vi "log analysis_gps.vi"() -> ()   [LabVIEW 2019] (continued)
\tsystem status\tnormal 2 28.000000 0 0\trobot status\t300.742789\t57.868654\t10.465800\t0.003841\t1.974526\t-29.727465\t0.303000\t-0.016000\n\t\n15:24:51.1\tlog_raw\tgps_raw\t#INSPVAXA,USB3,0,50.0,FINESTEERING,2107,282309.100,02000000,471d,15824;INS_ALIGNMENT_COMPLETE,INS_RTKFIXED,37.37065087449,126.72423169405,10.4716,22.3000,-0.1818,0.2462,0.0157,-0.101661617,1.756669202,119.993193465,0.5316,0.3505,0.6792,0.1345,0.1096,0.0793,0.1439,0.1491,4.9301,0f000001,0*2fa2c19e\n\tsystem status\tnormal 2 28.000000 0 0\trobot status\t300.864286\t57.781823\t10.471600\t-0.101662\t1.756669\t-29.993193\t0.301000\t-0.019000\n\t\n15:24:51.6\tlog_raw\tgps_raw\t#INSPVAXA,USB3,0,50.5,FINESTEERING,2107,282309.600,02000000,471d,15824;INS_ALIGNMENT_COMPLETE,INS_RTKFIXED,37.37065005438,126.72423301384,10.4771,22.3000,-0.1715,0.2318,0.0129,-0.072761707,1.702932866,120.296688789,0.5316,0.3505,0.6792,0.1345,0.1096,0.0793,0.1439,0.1491,4.9301,0f000001,0*35eea818\n\tsystem status\tnormal 2 28.000000 0 0\trobot status\t300.981191\t57.690799\t10.477100\t-0.072762\t1.702933\t-30.296689\t0.299000\t-0.017000\n\t\n15:24:52.1\tlog_raw\tgps_raw\t#DUALANTENNAHEADINGA,USB3,0,50.0,FINESTEERING,2107,282310.100,02000000,d426,15824;INSUFFICIENT_OBS,NONE,0.000000000,0.000000000,0.000000000,0.0,0.000000000,0.000000000,\"\",0,0,0,0,00,00,00,00*14cc2e90\n\tsystem status\tnormal 2 28.000000 0 0\trobot status\t301.096541\t57.598411\t10.483200\t0.061278\t1.632933\t-30.590921\t0.298000\t-0.016000\n\t\n15:24:52.6\tlog_raw\tgps_raw\t#INSPVAXA,USB3,0,50.0,FINESTEERING,2107,282310.600,02000000,471d,15824;INS_ALIGNMENT_COMPLETE,INS_RTKFIXED,37.37064838288,126.72423565428,10.4879,22.3000,-0.1825,0.2221,0.0118,0.275691228,1.663027619,120.773343582,0.5316,0.3505,0.6792,0.1345,0.1096,0.0793,0.1439,0.1491,4.9301,0f000001,0*997564fa\n\tsystem status\tnormal 2 28.000000 0 0\trobot status\t301.215077\t57.505280\t10.487900\t0.275691\t1.663028\t-30.773344\t0.300000\t-0.012000\n\t\n15:24:53.1\tlog_raw\tgps_raw\t#DUALANTENNAHEADINGA,USB3,0,46.0,FINESTEERING,2107,282311.100,02000000,d426,15824;SOL_COMPUTED,NARROW_FLOAT,-1.000000000,117.813430786,-36.691406250,0.0,360.000000000,180.000000000,\"631T\",17,7,7,6,04,00,20,03*31d6dfd5\n\tsystem status\tnormal 2 28.000000 0 0\trobot status\t301.329857\t57.414343\t10.492200\t0.192572\t1.804077\t-31.004968\t0.300000\t-0.009000\n\t\n15:24:53.6\tlog_raw\tgps_raw\t#DUALANTENNAHEADINGA,USB3,0,46.0,FINESTEERING,2107,282311.600,02000000,d426,15824;SOL_COMPUTED,NARROW_FLOAT,-1.000000000,120.262771606,-39.374176025,0.0,360.000000000,180.000000000,\"631T\",18,7,7,5,04,00,20,03*970c933d\n\tsystem status\tnormal 2 28.000000 0 0\trobot status\t301.442602\t57.321734\t10.497200\t0.226704\t1.873089\t-31.248181\t0.301000\t-0.010000\n\t\n15:24:54.1\tlog_raw\tgps_raw\t#INSPVAXA,USB3,0,48.5,FINESTEERING,2107,282312.100,02000000,471d,15824;INS_ALIGNMENT_COMPLETE,INS_RTKFIXED,37.37064587490,126.72423949786,10.5026,22.3000,-0.1922,0.2292,0.0073,0.477048241,1.745843480,121.477542384,0.5806,0.3850,0.7206,0.1397,0.1125,0.0814,0.1439,0.1495,4.9286,0f000001,0*cdf8ddfc\n\tsystem status\tnormal 2 28.000000 0 0\trobot status\t301.555535\t57.226921\t10.502600\t0.477048\t1.745843\t-31.477542\t0.299000\t-0.001000\n\t\n15:24:54.6\tlog_raw\tgps_raw\t#DUALANTENNAHEADINGA,USB3,0,48.5,FINESTEERING,2107,282312.600,02000000,d426,15824;INSUFFICIENT_OBS,NONE,0.000000000,0.000000000,0.000000000,0.0,0.000000000,0.000000000,\"\",0,0,0,0,00,00,00,00*914fc627\n\tsystem status\tnormal 2 28.100000 0 0\trobot status\t301.668360\t57.139659\t10.506800\t0.443490\t1.749413\t-31.695525\t0.299000\t0.005000\n\t\n15:24:55.1\tlog_raw\tgps_raw\t#INSPVAXA,USB3,0,48.0,FINESTEERING,2107,282313.100,02000000,471d,15824;INS_ALIGNMENT_COMPLETE,INS_RTKFIXED,37.37064429153,126.72424202455,10.5097,22.3000,-0.1991,0.2355,-0.0061,0.301334832,1.691394524,121.905200566,0.5806,0.3850,0.7206,0.1397,0.1125,0.0814,0.1439,0.1495,4.9286,0f000001,0*1a642130\n\tsystem status\tnormal 2 28.100000 0 0\trobot status\t301.779345\t57.051183\t10.509700\t0.301335\t1.691395\t-31.905201\t0.295000\t0.004000\n\t\n15:24:55.6\tlog_raw\tgps_raw\t#DUALANTENNAHEADINGA,USB3,0,48.0,FINESTEERING,2107,282313.600,02000000,d426,15824;INSUFFICIENT_OBS,NONE,0.000000000,0.000000000,0.000000000,0.0,0.000000000,0.000000000,\"\",0,0,0,0,00,00,00,00*80ae0999\n\tsystem status\tnormal 2 28.100000 0 0\trobot status\t301.892959\t56.952693\t10.513100\t0.176842\t1.740351\t-31.947906\t0.299000\t0.002000\n\t\n15:24:56.1\tlog_raw\tgps_raw\t#DUALANTENNAHEADINGA,USB3,0,48.0,FINESTEERING,2107,282314.100,02000000,d426,15824;SOL_COMPUTED,NARROW_FLOAT,-1.000000000,134.357482910,-58.416107178,0.0,360.000000000,180.000000000,\"631T\",15,6,6,5,04,00,20,03*a0098d17\n\tsystem status\tnormal 2 28.000000 0 0\trobot status\t302.007556\t56.850426\t10.516100\t0.276136\t1.780123\t-31.941139\t0.297000\t0.012000\n\t\n15:24:56.6\tlog_raw\tgps_raw\t#INSPVAXA,USB3,0,53.0,FINESTEERING,2107,282314.600,02000000,471d,15824;INS_ALIGNMENT_COMPLETE,INS_RTKFIXED,37.37064155403,126.72424590503,10.5186,22.3000,-0.2085,0.2358,0.0044,0.281854568,1.880117721,121.982291751,0.5806,0.3850,0.7206,0.1397,0.1125,0.0814,0.1439,0.1495,4.9286,0f000001,0*a4c93626\n\tsystem status\tnormal 2 28.000000 0 0\trobot status\t302.123071\t56.747350\t10.518600\t0.281855\t1.880118\t-31.982292\t0.296000\t0.011000\n\t\n15:24:57.1\tlog_raw\tgps_raw\t#DUALANTENNAHEADINGA,USB3,0,51.5,FINESTEERING,2107,282315.100,02000000,d426,15824;INSUFFICIENT_OBS,NONE,0.000000000,0.000000000,0.000000000,0.0,0.000000000,0.000000000,\"\",0,0,0,0,00,00,00,00*fb6d87b7\n\tsystem status\tnormal 2 28.100000 0 0\trobot status\t302.241242\t56.647460\t10.522500\t0.119522\t1.963027\t-31.987083\t0.304000\t0.000000\n\t\n15:24:57.6\tlog_raw\tgps_raw\t#DUALANTENNAHEADINGA,USB3,0,51.5,FINESTEERING,2107,282315.600,02000000,d426,15824;INSUFFICIENT_OBS,NONE,0.000000000,0.000000000,0.000000000,0.0,0.000000000,0.000000000,\"\",0,0,0,0,00,00,00,00*5226e786\n\tsystem status\tnormal 2 28.000000 0 0\trobot status\t302.361937\t56.570829\t10.531100\t-0.048140\t2.044606\t-31.974710\t0.298000\t0.005000\n\t\n15:24:58.1\tlog_raw\tgps_raw\t#DUALANTENNAHEADINGA,USB3,0,48.0,FINESTEERING,2107,282316.100,02000000,d426,15824;SOL_COMPUTED,NARROW_FLOAT,-1.000000000,136.040298462,-67.713562012,0.0,360.000000000,180.000000000,\"631T\",17,7,7,5,04,00,20,03*78f64e13\n\tsystem status\tnormal 2 28.000000 0 0\trobot status\t302.481985\t56.490419\t10.539400\t-0.282302\t1.973915\t-31.798281\t0.368000\t-0.099000\n\t\n15:24:58.6\tlog_raw\tgps_raw\t#DUALANTENNAHEADINGA,USB3,0,48.0,FINESTEERING,2107,282316.600,02000000,d426,15824;SOL_COMPUTED,NARROW_FLOAT,-1.000000000,134.914855957,-67.706207275,0.0,360.000000000,180.000000000,\"631T\",16,7,7,5,04,00,20,03*7ca473fa\n\tsystem status\tnormal 2 28.000000 0 0\trobot status\t302.597622\t56.388381\t10.542900\t-0.264401\t2.039387\t-31.436146\t0.256000\t0.072000\n\t\n15:24:59.1\tlog_raw\tgps_raw\t#DUALANTENNAHEADINGA,USB3,0,48.0,FINESTEERING,2107,282317.100,02000000,d426,15824;SOL_COMPUTED,L1_FLOAT,-1.000000000,88.879760742,-51.174438477,0.0,360.000000000,180.000000000,\"631T\",15,6,6,3,04,00,20,01*bfb98121\n\tsystem status\tnormal 2 27.900000 0 0\trobot status\t302.712943\t56.290986\t10.546800\t-0.242492\t1.961674\t-31.012950\t0.317000\t-0.003000\n\t\n15:24:59.6\tlog_raw\tgps_raw\t#DUALANTENNAHEADINGA,USB3,0,50.0,FINESTEERING,2107,282317.600,02000000,d426,15824;SOL_COMPUTED,L1_FLOAT,-1.000000000,88.347457886,-50.822692871,0.0,360.000000000,180.000000000,\"631T\",15,6,6,3,04,00,20,01*5e456794\n\tsystem status\tnormal 2 27.900000 0 0\trobot status\t302.824447\t56.222080\t10.554900\t-0.396426\t2.099924\t-30.552622\t0.307000\t0.004000\n\t\n15:25:00.1\tlog_raw\tgps_raw\t#DUALANTENNAHEADINGA,USB3,0,50.0,FINESTEERING,2107,282318.100,02000000,d426,15824;INSUFFICIENT_OBS,NONE,0.000000000,0.000000000,0.000000000,0.0,0.000000000,0.000000000,\"\",0,0,0,0,00,00,00,00*a99f8f24\n\tsystem status\tnormal 2 27.900000 0 0\trobot status\t302.938938\t56.151661\t10.562300\t-0.544114\t2.007345\t-30.070120\t0.286000\t0.028000\n\t\n15:25:00.6\tlog_raw\tgps_raw\t#DUALANTENNAHEADINGA,USB3,0,51.5,FINESTEERING,2107,282318.600,02000000,d426,15824;INSUFFICIENT_OBS,NONE,0.000000000,0.000000000,0.000000000,0.0,0.000000000,0.000000000,\"\",0,0,0,0,00,00,00,00*4bce61fe\n\tsystem status\tnormal 2 27.900000 0 0\trobot status\t303.057315\t56.072035\t10.568200\t-0.724455\t1.935661\t-29.531309\t0.228000\t0.116000\n\t\n15:25:01.1\tlog_raw\tgps_raw\t#DUALANTENNAHEADINGA,USB3,0,51.5,FINESTEERING,2107,282319.100,02000000,d426,15824;SOL_COMPUTED,NARROW_FLOAT,-1.000000000,152.278427124,-75.170898438,0.0,360.000000000,65.870956421,\"631T\",16,7,7,5,04,00,20,03*bcd3d891\n\tsystem status\tnormal 2 27.900000 0 0\trobot status\t303.173391\t55.989421\t10.573500\t-0.593101\t2.053140\t-29.157767\t0.206000\t0.136000\n\t\n15:25:01.6\tlog_raw\tgps_raw\t#DUALANTENNAHEADINGA,USB3,0,52.5,FINESTEERING,2107,282319.600,02000000,d426,15824;SOL_COMPUTED,NARROW_FLOAT,-1.000000000,152.142578125,-75.197906494,0.0,360.000000000,65.816017151,\"631T\",16,7,7,5,04,00,20,03*ee26bdb3\n\tsystem status\tnormal 2 27.900000 0 0\trobot status\t303.292783\t55.893004\t10.575700\t-0.534570\t1.919826\t-28.776034\t0.366000\t-0.103000\n\t\n15:25:02.1\tlog_raw\tgps_raw\t#DUALANTENNAHEADINGA,USB3,0,46.0,FINESTEERING,2107,282320.100,02000000,d426,15824;SOL_COMPUTED,NARROW_FLOAT,-1.000000000,137.905578613,-56.183776855,0.0,360.000000000,180.000000000,\"631T\",15,6,6,5,04,00,20,03*ad4a7336\n\tsystem status\tnormal 2 28.000000 0 0\trobot status\t303.413887\t55.800073\t10.578400\t-0.652078\t1.747605\t-28.605131\t0.246000\t0.075000\n\t\n15:25:02.6\tlog_raw\tgps_raw\t#DUALANTENNAHEADINGA,USB3,0,46.0,FINESTEERING,2107,282320.600,02000000,d426,15824;SOL_COMPUTED,NARROW_FLOAT,-1.000000000,138.732131958,-57.118835449,0.0,360.000000000,180.000000000,\"631T\",15,6,6,5,04,00,20,03*b657a1f8\n\tsystem status\tnormal 2 28.000000 0 0\trobot status\t303.533302\t55.728567\t10.584100\t-0.671421\t1.687664\t-28.425331\t0.242000\t0.088000\n\t\n15:25:03.1\tlog_raw\tgps_raw\t#DUALANTENNAHEADINGA,USB3,0,46.0,FINESTEERING,2107,282321.100,02000000,d426,15824;SOL_COMPUTED,NARROW_FLOAT,-1.000000000,138.171997070,-47.447601318,0.0,360.000000000,180.000000000,\"631T\",17,6,6,5,04,00,20,03*1bd00597\n\tsystem status\tnormal 2 28.000000 0 0\trobot status\t303.652575\t55.655599\t10.590200\t-0.618305\t1.582837\t-28.345592\t0.281000\t0.026000\n\t\n15:25:03.6\tlog_raw\tgps_raw\t#DUALANTENNAHEADINGA,USB3,0,50.0,FINESTEERING,2107,282321.600,02000000,d426,15824;SOL_COMPUTED,NARROW_FLOAT,-1.000000000,138.598281860,-47.134765625,0.0,360.000000000,180.000000000,\"631T\",17,6,6,5,04,00,20,03*7418056f\n\tsystem status\tnormal 2 28.000000 0 0\trobot status\t303.771153\t55.579183\t10.594700\t-0.578727\t1.493465\t-28.246087\t0.340000\t-0.070000\n\t\n15:25:04.1\tlog_raw\tgps_raw\t#DUALANTENNAHEADINGA,USB3,0,50.0,FINESTEERING,2107,282322.100,02000000,d426,15824;SOL_COMPUTED,NARROW_FLOAT,-1.000000000,138.887161255,-70.719177246,0.0,360.000000000,133.361663818,\"631T\",17,7,7,5,04,00,20,03*5d30d365\n\tsystem status\tnormal 2 28.100000 0 0\trobot status\t303.890807\t55.500835\t10.598600\t-0.554636\t1.420103\t-28.284679\t0.298000\t-0.006000\n\t\n15:25:04.6\tlog_raw\tgps_raw\t#DUALANTENNAHEADINGA,USB3,0,50.5,FINESTEERING,2107,282322.600,02000000,d426,15824;SOL_COMPUTED,NARROW_FLOAT,-1.000000000,137.188095093,-70.605590820,0.0,360.000000000,140.173141479,\"631T\",17,7,7,5,04,00,20,02*f8e674e7\n\tsystem status\tnormal 2 28.000000 0 0\trobot status\t304.007206\t55.423299\t10.602300\t-0.567177\t1.389661\t-28.394288\t0.300000\t-0.013000\n\t\n15:25:05.1\tlog_raw\tgps_raw\t#DUALANTENNAHEADINGA,USB3,0,50.5,FINESTEERING,2107,282323.100,02000000,d426,15824;INSUFFICIENT_OBS,NONE,0.000000000,0.000000000,0.000000000,0.0,0.000000000,0.000000000,\"\",0,0,0,0,00,00,00,00*ed7be7e8\n\tsystem status\tnormal 2 28.000000 0 0\trobot status\t304.122143\t55.344457\t10.604600\t-0.434721\t1.206100\t-28.438230\t0.297000\t-0.019000\n\t\n15:25:05.6\tlog_raw\tgps_raw\t#DUALANTENNAHEADINGA,USB3,0,51.0,FINESTEERING,2107,282323.600,02000000,d426,15824;INSUFFICIENT_OBS,NONE,0.000000000,0.000000000,0.000000000,0.0,0.000000000,0.000000000,\"\",0,0,0,0,00,00,00,00*0f2a0932\n\tsystem status\tnormal 2 28.100000 0 0\trobot status\t304.235843\t55.267053\t10.605000\t-0.412343\t1.239583\t-28.504935\t0.294000\t-0.023000\n\t\n15:25:06.1\tlog_raw\tgps_raw\t#DUALANTENNAHEADINGA,USB3,0,51.0,FINESTEERING,2107,282324.100,02000000,d426,15824;INSUFFICIENT_OBS,NONE,0.000000000,0.000000000,0.000000000,0.0,0.000000000,0.000000000,\"\",0,0,0,0,00,00,00,00*2d8ea6a2\n\tsystem status\tnormal 2 28.000000 0 0\trobot status\t304.351241\t55.185294\t10.605200\t-0.412073\t1.305479\t-28.610817\t0.300000\t-0.015000\n\t\n15:25:06.6\tlog_raw\tgps_raw\t#DUALANTENNAHEADINGA,USB3,0,51.5,FINESTEERING,2107,282324.600,02000000,d426,15824;INSUFFICIENT_OBS,NONE,0.000000000,0.000000000,0.000000000,0.0,0.000000000,0.000000000,\"\",0,0,0,0,00,00,00,00*6f36fe3b\n\tsystem status\tnormal 2 28.000000 0 0\trobot status\t304.465831\t55.091737\t10.605100\t-0.396944\t1.414382\t-28.827248\t0.298000\t-0.017000\n\t\n15:25:07.1\tlog_raw\tgps_raw\t#DUALANTENNAHEADINGA,USB3,0,51.5,FINESTEERING,2107,282325.100,02000000,d426,15824;SOL_COMPUTED,NARROW_FLOAT,-1.000000000,140.911849976,-56.769714355,0.0,360.000000000,180.000000000,\"631T\",16,6,6,5,04,00,20,03*7a8a24a8\n\tsystem status\tnormal 2 28.000000 0 0\trobot status\t304.584903\t54.993442\t10.604900\t-0.316373\t1.496680\t-29.102629\t0.299000\t-0.025000\n\t\n15:25:07.6\tlog_raw\tgps_raw\t#DUALANTENNAHEADINGA,USB3,0,52.0,FINESTEERING,2107,282325.600,02000000,d426,15824;SOL_COMPUTED,NARROW_FLOAT,-1.000000000,140.545684814,-57.778442383,0.0,360.000000000,180.000000000,\"631T\",15,6,6,5,04,00,20,03*6799af52\n\tsystem status\tnormal 2 28.000000 0 0\trobot status\t304.705154\t54.894059\t10.604300\t-0.443336\t1.624461\t-29.353029\t0.296000\t-0.011000\n\t\n15:25:08.1\tlog_raw\tgps_raw\t#DUALANTENNAHEADINGA,USB3,0,51.5,FINESTEERING,2107,282326.100,02000000,d426,15824;INSUFFICIENT_OBS,NONE,0.000000000,0.000000000,0.000000000,0.0,0.000000000,0.000000000,\"\",0,0,0,0,00,00,00,00*e9297667\n\tsystem status\tnormal 2 28.000000 0 0\trobot status\t304.821221\t54.801549\t10.605500\t-0.522015\t1.704805\t-29.612871\t0.302000\t-0.019000\n\t\n15:25:08.6\tlog_raw\tgps_raw\t#DUALANTENNAHEADINGA,USB3,0,51.5,FINESTEERING,2107,282326.600,02000000,d426,15824;INSUFFICIENT_OBS,NONE,0.000000000,0.000000000,0.000000000,0.0,0.000000000,0.000000000,\"\",0,0,0,0,00,00,00,00*40621656\n\tsystem status\tnormal 2 28.000000 0 0\trobot status\t304.937471\t54.740446\t10.612400\t-0.542865\t1.810762\t-29.827775\t0.300000\t-0.006000\n\t\n15:25:09.1\tlog_raw\tgps_raw\t#DUALANTENNAHEADINGA,USB3,0,50.5,FINESTEERING,2107,282327.100,02000000,d426,15824;SOL_COMPUTED,NARROW_FLOAT,-1.000000000,125.369018555,-45.270568848,0.0,360.000000000,180.000000000,\"631T\",15,6,6,5,04,00,20,03*24996260\n\tsystem status\tnormal 2 28.000000 0 0\trobot status\t305.052718\t54.671777\t10.617100\t-0.538561\t1.705950\t-30.003874\t0.298000\t-0.002000\n\t\n15:25:09.6\tlog_raw\tgps_raw\t#DUALANTENNAHEADINGA,USB3,0,50.5,FINESTEERING,2107,282327.600,02000000,d426,15824;SOL_COMPUTED,NARROW_FLOAT,-1.000000000,125.215858459,-46.956237793,0.0,360.000000000,180.000000000,\"631T\",16,6,6,5,04,00,20,03*d17be84f\n\tsystem status\tnormal 2 28.000000 0 0\trobot status\t305.169009\t54.574272\t10.617100\t-0.762339\t1.572300\t-30.237669\t0.298000\t-0.009000\n\t\n15:25:10.1\tlog_raw\tgps_raw\t#DUALANTENNAHEADINGA,USB3,0,50.5,FINESTEERING,2107,282328.100,02000000,d426,15824;INSUFFICIENT_OBS,NONE,0.000000000,0.000000000,0.000000000,0.0,0.000000000,0.000000000,\"\",0,0,0,0,00,00,00,00*856e5927\n\tsystem status\tnormal 2 28.000000 0 0\trobot status\t305.281444\t54.481832\t10.618900\t-0.831746\t1.481777\t-30.539576\t0.302000\t-0.016000\n\t\n15:25:10.6\tlog_raw\tgps_raw\t#DUALANTENNAHEADINGA,USB3,0,51.5,FINESTEERING,2107,282328.600,02000000,d426,15824;INSUFFICIENT_OBS,NONE,0.000000000,0.000000000,0.000000000,0.0,0.000000000,0.000000000,\"\",0,0,0,0,00,00,00,00*8ccc8f55\n\tsystem status\tnormal 2 28.000000 0 0\trobot status\t305.395322\t54.419135\t10.626700\t-1.019045\t1.320970\t-30.834865\t0.294000\t-0.012000\n\t\n15:25:11.1\tlog_raw\tgps_raw\t#DUALANTENNAHEADINGA,USB3,0,51.5,FINESTEERING,2107,282329.100,02000000,d426,15824;SOL_COMPUTED,L1_FLOAT,-1.000000000,81.258789063,-50.005187988,0.0,360.000000000,180.000000000,\"631T\",16,6,6,3,04,00,20,01*7dc2aa1f\n\tsystem status\tnormal 2 28.000000 0 0\trobot status\t305.510325\t54.347562\t10.632800\t-1.023114\t1.125484\t-31.050463\t0.300000\t-0.006000\n\t\n15:25:11.6\tlog_raw\tgps_raw\t#DUALANTENNAHEADINGA,USB3,0,52.0,FINESTEERING,2107,282329.600,02000000,d426,15824;SOL_COMPUTED,L1_FLOAT,-1.000000000,80.095443726,-49.685882568,0.0,360.000000000,180.000000000,\"631T\",16,6,6,4,04,00,20,03*d7163941\n\tsystem status\tnormal 2 28.000000 0 0\trobot status\t305.620625\t54.252693\t10.632800\t-1.118178\t1.147397\t-31.279123\t0.296000\t-0.001000\n\t\n15:25:12.1\tlog_raw\tgps_raw\t\tsystem status\tnormal 2 28.000000 0 0\trobot status\t305.732891\t54.160003\t10.633600\t-1.193297\t1.211031\t-31.471931\t0.296000\t-0.003000\n\t\n15:25:12.6\tlog_raw\tgps_raw\t\tsystem status\tnormal 2 28.000000 0 0\trobot status\t305.846846\t54.092869\t10.641800\t-1.220329\t1.272056\t-31.645631\t0.299000\t-0.003000\n\t\n15:25:13.1\tlog_raw\tgps_raw\t#DUALANTENNAHEADINGA,USB3,0,52.0,FINESTEERING,2107,282331.100,02000000,d426,15824;INSUFFICIENT_OBS,NONE,0.000000000,0.000000000,0.000000000,0.0,0.000000000,0.000000000,\"\",0,0,0,0,00,00,00,00*4750fa4c\n\tsystem status\tnormal 2 28.000000 0 0\trobot status\t305.958475\t54.021236\t10.648300\t-1.360665\t1.228088\t-31.866711\t0.294000\t0.004000\n\t\n15:25:13.6\tlog_raw\tgps_raw\t\tsystem status\tnormal 2 28.000000 0 0\trobot status\t306.064764\t53.926766\t10.647700\t-1.290973\t1.326680\t-32.101043\t0.296000\t-0.001000\n\t\n15:25:14.1\tlog_raw\tgps_raw\t#DUALANTENNAHEADINGA,USB3,0,51.5,FINESTEERING,2107,282332.100,02000000,d426,15824;INSUFFICIENT_OBS,NONE,0.000000000,0.000000000,0.000000000,0.0,0.000000000,0.000000000,\"\",0,0,0,0,00,00,00,00*43ae011b\n\tsystem status\tnormal 2 28.000000 0 0\trobot status\t306.168708\t53.833607\t10.646700\t-1.358548\t1.265281\t-32.328757\t0.296000\t0.008000\n\t\n15:25:14.6\tlog_raw\tgps_raw\t\tsystem status\tnormal 2 28.000000 0 0\trobot status\t306.273334\t53.738935\t10.645800\t-1.442913\t1.039902\t-32.541755\t0.302000\t0.006000\n\t\n15:25:15.1\tlog_raw\tgps_raw\t#DUALANTENNAHEADINGA,USB3,0,51.5,FINESTEERING,2107,282333.100,02000000,d426,15824;INSUFFICIENT_OBS,NONE,0.000000000,0.000000000,0.000000000,0.0,0.000000000,0.000000000,\"\",0,0,0,0,00,00,00,00*b9bcf60d\n\tsystem status\tnormal 2 28.000000 0 0\trobot status\t306.381214\t53.649615\t10.646500\t-1.625830\t0.971888\t-32.675869\t0.297000\t0.002000\n\t\n15:25:15.6\tlog_raw\tgps_raw\t#DUALANTENNAHEADINGA,USB3,0,53.0,FINESTEERING,2107,282333.600,02000000,d426,15824;INSUFFICIENT_OBS,NONE,0.000000000,0.000000000,0.000000000,0.0,0.000000000,0.000000000,\"\",0,0,0,0,00,00,00,00*61a6c453\n\tsystem status\tnormal 2 28.000000 0 0\trobot status\t306.504139\t53.584085\t10.655000\t-1.672742\t0.985085\t-32.728934\t0.303000\t0.016000\n\t\n15:25:16.1\tlog_raw\tgps_raw\t\tsystem status\tnormal 2 28.000000 0 0\trobot status\t306.629194\t53.512535\t10.663000\t-1.579739\t0.946344\t-32.854770\t0.302000\t-0.002000\n\t\n15:25:16.6\tlog_raw\tgps_raw\t#DUALANTENNAHEADINGA,USB3,0,50.5,FINESTEERING,2107,282334.600,02000000,d426,15824;INSUFFICIENT_OBS,NONE,0.000000000,0.000000000,0.000000000,0.0,0.000000000,0.000000000,\"\",0,0,0,0,00,00,00,00*3bf1efde\n\tsystem status\tnormal 2 28.000000 0 0\trobot status\t306.744397\t53.430829\t10.669500\t-1.580379\t0.887830\t-32.888651\t0.297000\t-0.001000\n\t\n15:25:17.1\tlog_raw\tgps_raw\t\tsystem status\tnormal 2 28.100000 0 0\trobot status\t306.858635\t53.348849\t10.675600\t-1.572290\t1.060751\t-32.929507\t0.296000\t0.000000\n\t\n15:25:17.6\tlog_raw\tgps_raw\t#DUALANTENNAHEADINGA,USB3,0,53.0,FINESTEERING,2107,282335.600,02000000,d426,15824;SOL_COMPUTED,NARROW_FLOAT,-1.000000000,106.698776245,-65.583465576,0.0,360.000000000,180.000000000,\"631T\",15,7,7,5,04,00,20,03*5d10cc48\n\tsystem status\tnormal 2 28.000000 0 0\trobot status\t306.969032\t53.266713\t10.683200\t-1.705061\t1.145161\t-32.913171\t0.298000\t0.007000\n\t\n15:25:18.1\tlog_raw\tgps_raw\t#DUALANTENNAHEADINGA,USB3,0,52.0,FINESTEERING,2107,282336.100,02000000,d426,15824;SOL_COMPUTED,L1_FLOAT,-1.000000000,75.314010620,-41.766326904,0.0,360.000000000,180.000000000,\"631T\",16,6,6,3,04,00,20,01*05518b35\n\tsystem status\tnormal 2 28.000000 0 0\trobot status\t307.082809\t53.181237\t10.691100\t-1.592914\t1.089623\t-32.880837\t0.264000\t0.059000\n\t\n15:25:18.6\tlog_raw\tgps_raw\t#DUALANTENNAHEADINGA,USB3,0,52.0,FINESTEERING,2107,282336.600,02000000,d426,15824;SOL_COMPUTED,L1_FLOAT,-1.000000000,75.472106934,-40.715057373,0.0,360.000000000,180.000000000,\"631T\",16,6,6,3,04,00,20,01*06f451b5\n\tsystem status\tnormal 2 28.000000 0 0\trobot status\t307.193484\t53.097798\t10.698000\t-1.485206\t1.157360\t-32.808638\t0.337000\t-0.065000\n\t\n15:25:19.1\tlog_raw\tgps_raw\t#INSPVAXA,USB3,0,49.0,FINESTEERING,2107,282337.150,02000000,471d,15824;INS_ALIGNMENT_COMPLETE,INS_RTKFIXED,37.37060784122,126.72430452808,10.7036,22.3000,-0.1718,0.2091,0.0001,-1.383604006,1.084294313,122.725543764,0.4496,0.3001,0.5813,0.1247,0.1017,0.0764,0.1414,0.1471,4.9509,0f000001,0*50e8e3f0\n\tsystem status\tnormal 2 28.000000 0 0\trobot status\t307.315805\t53.005558\t10.703600\t-1.383604\t1.084294\t-32.725544\t0.280000\t0.025000\n\t\n15:25:19.6\tlog_raw\tgps_raw\t\tsystem status\tnormal 2 28.000000 0 0\trobot status\t307.416498\t52.929659\t10.708000\t-1.302899\t1.013526\t-32.649985\t0.352000\t-0.086000\n\t\n15:25:20.1\tlog_raw\tgps_raw\t#DUALANTENNAHEADINGA,USB3,0,49.0,FINESTEERING,2107,282338.100,02000000,d426,15824;SOL_COMPUTED,L1_FLOAT,-1.000000000,82.313255310,23.154996872,0.0,360.000000000,180.000000000,\"631T\",16,5,5,3,04,00,20,01*91a11998\n\tsystem status\tnormal 2 28.000000 0 0\trobot status\t307.526938\t52.846677\t10.712500\t-1.224950\t0.927334\t-32.483439\t0.289000\t0.008000\n\t\n15:25:20.6\tlog_raw\tgps_raw\t\tsystem status\tnormal 2 28.000000 0 0\trobot status\t307.628954\t52.764694\t10.714300\t-1.046370\t0.891520\t-32.240885\t0.243000\t0.080000\n\t\n15:25:21.1\tlog_raw\tgps_raw\t#DUALANTENNAHEADINGA,USB3,0,50.5,FINESTEERING,2107,282339.100,02008000,d426,15824;INSUFFICIENT_OBS,NONE,0.000000000,0.000000000,0.000000000,0.0,0.000000000,0.000000000,\"\",0,0,0,0,00,00,00,00*9d87d1bd\n\tsystem status\tnormal 2 28.000000 0 0\trobot status\t307.734345\t52.683097\t10.716500\t-0.921301\t0.937395\t-32.102084\t0.385000\t-0.119000\n\t\n15:25:21.6\tlog_raw\tgps_raw\t#INSPVAXA,USB3,0,52.0,FINESTEERING,2107,282339.650,02008000,471d,15824;INS_ALIGNMENT_COMPLETE,INS_RTKFIXED,37.37060410309,126.72431070985,10.7187,22.3000,-0.1560,0.2044,-0.0028,-0.834208822,1.087221031,121.798208463,0.4988,0.3371,0.6091,0.1298,0.1043,0.0790,0.1415,0.1476,4.9532,0f000001,0*1343af04\n\tsystem status\tnormal 2 28.000000 0 0\trobot status\t307.863376\t52.590663\t10.718700\t-0.834209\t1.087221\t-31.798208\t0.269000\t0.059000\n\t\n15:25:22.1\tlog_raw\tgps_raw\t#DUALANTENNAHEADINGA,USB3,0,50.5,FINESTEERING,2107,282340.100,02008000,d426,15824;INSUFFICIENT_OBS,NONE,0.000000000,0.000000000,0.000000000,0.0,0.000000000,0.000000000,\"\",0,0,0,0,00,00,00,00*7b9cfbae\n\tsystem status\tnormal 2 28.000000 0 0\trobot status\t307.968248\t52.516400\t10.720000\t-0.765356\t0.932327\t-31.608754\t0.295000\t0.000000\n\t\n15:25:22.6\tlog_raw\tgps_raw\t#DUALANTENNAHEADINGA,USB3,0,50.5,FINESTEERING,2107,282340.600,02008000,d426,15824;INSUFFICIENT_OBS,NONE,0.000000000,0.000000000,0.000000000,0.0,0.000000000,0.000000000,\"\",0,0,0,0,00,00,00,00*d2d79b9f\n\tsystem status\tnormal 2 28.000000 0 0\trobot status\t308.073059\t52.439538\t10.720700\t-0.779600\t0.914294\t-31.399334\t0.366000\t-0.090000\n\t\n15:25:23.1\tlog_raw\tgps_raw\t#DUALANTENNAHEADINGA,USB3,0,50.5,FINESTEERING,2107,282341.100,02008000,d426,15824;SOL_COMPUTED,NARROW_FLOAT,-1.000000000,114.279808044,-67.503875732,0.0,360.000000000,180.000000000,\"631T\",19,7,7,5,04,00,20,03*2721f886\n\tsystem status\tnormal 2 28.100000 0 0\trobot status\t308.175756\t52.364301\t10.721900\t-0.721086\t1.080346\t-31.232334\t0.297000\t0.003000\n\t\n15:25:23.6\tlog_raw\tgps_raw\t#INSPVAXA,USB3,0,51.0,FINESTEERING,2107,282341.650,02008000,471d,15824;INS_ALIGNMENT_COMPLETE,INS_RTKFIXED,37.37060132873,126.72431550625,10.7234,22.3000,-0.1474,0.2047,-0.0035,-0.652632688,1.321187419,121.044830235,0.4988,0.3371,0.6091,0.1298,0.1043,0.0790,0.1415,0.1476,4.9532,0f000001,0*64211db3\n\tsystem status\tnormal 2 28.000000 0 0\trobot status\t308.288233\t52.282736\t10.723400\t-0.652633\t1.321187\t-31.044830\t0.313000\t-0.009000\n\t\n15:25:24.1\tlog_raw\tgps_raw\t#DUALANTENNAHEADINGA,USB3,0,51.0,FINESTEERING,2107,282342.100,02008000,d426,15824;INSUFFICIENT_OBS,NONE,0.000000000,0.000000000,0.000000000,0.0,0.000000000,0.000000000,\"\",0,0,0,0,00,00,00,00*1fd29d28\n\tsystem status\tnormal 2 28.000000 0 0\trobot status\t308.385379\t52.212101\t10.725700\t-0.538350\t1.326991\t-31.017273\t0.264000\t0.059000\n\t\n15:25:24.6\tlog_raw\tgps_raw\t#DUALANTENNAHEADINGA,USB3,0,53.0,FINESTEERING,2107,282342.600,02008000,d426,15824;INSUFFICIENT_OBS,NONE,0.000000000,0.000000000,0.000000000,0.0,0.000000000,0.000000000,\"\",0,0,0,0,00,00,00,00*2c3b97de\n\tsystem status\tnormal 2 28.000000 0 0\trobot status\t308.519784\t52.118516\t10.733000\t-0.677844\t1.619004\t-30.960246\t0.256000\t0.064000\n\t\n15:25:25.1\tlog_raw\tgps_raw\t\tsystem status\tnormal 2 28.000000 0 0\trobot status\t308.651373\t52.028070\t10.740000\t-0.859266\t1.865383\t-30.849763\t0.284000\t0.016000\n\t\n15:25:25.6\tlog_raw\tgps_raw\t\tsystem status\tnormal 2 28.000000 0 0\trobot status\t308.758279\t51.953218\t10.742900\t-0.804322\t1.881980\t-30.789870\t0.254000\t0.076000\n\t\n15:25:26.1\tlog_raw\tgps_raw\t#INSPVAXA,USB3,0,54.0,FINESTEERING,2107,282344.150,02000000,471d,15824;INS_ALIGNMENT_COMPLETE,INS_RTKFIXED,37.37059762700,126.72432213612,10.7457,22.3000,-0.1412,0.2163,0.0072,-0.887257962,1.775723186,120.744197339,0.5693,0.3802,0.6775,0.1345,0.1064,0.0820,0.1423,0.1482,4.9577,0f000001,0*eda97082\n\tsystem status\tnormal 2 28.000000 0 0\trobot status\t308.875496\t51.871879\t10.745700\t-0.887258\t1.775723\t-30.744197\t0.295000\t0.009000\n\t\n15:25:26.6\tlog_raw\tgps_raw\t#INSPVAXA,USB3,0,54.0,FINESTEERING,2107,282344.650,02000000,471d,15824;INS_ALIGNMENT_COMPLETE,INS_RTKFIXED,37.37059696338,126.72432331213,10.7485,22.3000,-0.1428,0.2163,0.0073,-0.851471886,1.782877792,120.701591584,0.5693,0.3802,0.6775,0.1345,0.1064,0.0820,0.1423,0.1482,4.9577,0f000001,0*59042419\n\tsystem status\tnormal 2 28.000000 0 0\trobot status\t308.979665\t51.798224\t10.748500\t-0.851472\t1.782878\t-30.701592\t0.298000\t0.000000\n\t\n15:25:27.1\tlog_raw\tgps_raw\t#INSPVAXA,USB3,0,55.5,FINESTEERING,2107,282345.150,02000000,471d,15824;INS_ALIGNMENT_COMPLETE,INS_RTKFIXED,37.37059621025,126.72432460307,10.7527,22.3000,-0.1388,0.2123,-0.0024,-0.823739386,1.527099287,120.736340769,0.5930,0.3895,0.7245,0.1352,0.1094,0.0826,0.1432,0.1486,4.9599,0f000001,0*b8434a6e\n\tsystem status\tnormal 2 28.000000 0 0\trobot status\t309.094015\t51.714634\t10.752700\t-0.823739\t1.527099\t-30.736341\t0.299000\t-0.005000\n\t\n15:25:27.6\tlog_raw\tgps_raw\t#DUALANTENNAHEADINGA,USB3,0,55.5,FINESTEERING,2107,282345.600,02000000,d426,15824;SOL_COMPUTED,L1_FLOAT,-1.000000000,162.531326294,-26.929321289,0.0,360.000000000,180.000000000,\"631T\",14,5,5,5,04,00,20,03*11a6b9e7\n\tsystem status\tnormal 2 28.000000 0 0\trobot status\t309.215646\t51.620733\t10.761200\t-0.937395\t1.601352\t-30.730171\t0.301000\t0.000000\n\t\n15:25:28.1\tlog_raw\tgps_raw\t\tsystem status\tnormal 2 28.000000 0 0\trobot status\t309.348466\t51.517633\t10.770100\t-0.926327\t1.727833\t-30.729478\t0.298000\t-0.011000\n\t\n15:25:28.6\tlog_raw\tgps_raw\t#INSPVAXA,USB3,0,51.0,FINESTEERING,2107,282346.650,02000000,471d,15824;INS_ALIGNMENT_COMPLETE,INS_RTKFIXED,37.37059354728,126.72432896514,10.7808,22.3000,-0.1593,0.2217,0.0028,-1.002740448,1.844752135,120.714031734,0.5188,0.3373,0.6687,0.1274,0.1044,0.0789,0.1425,0.1477,4.9597,0f000001,0*e05fc804\n\tsystem status\tnormal 2 28.000000 0 0\trobot status\t309.480400\t51.419071\t10.780800\t-1.002740\t1.844752\t-30.714032\t0.302000\t0.000000\n\t\n15:25:29.1\tlog_raw\tgps_raw\t#INSPVAXA,USB3,0,53.5,FINESTEERING,2107,282347.150,02000000,471d,15824;INS_ALIGNMENT_COMPLETE,INS_RTKFIXED,37.37059272987,126.72433032061,10.7898,22.3000,-0.1653,0.2242,0.0071,-0.929787730,1.969126330,120.702008757,0.4813,0.3140,0.6303,0.1252,0.1036,0.0771,0.1422,0.1473,4.9596,0f000001,0*9ccf88c1\n\tsystem status\tnormal 2 28.000000 0 0\trobot status\t309.600465\t51.328347\t10.789800\t-0.929788\t1.969126\t-30.702009\t0.299000\t0.003000\n\t\n15:25:29.6\tlog_raw\tgps_raw\t#INSPVAXA,USB3,0,53.5,FINESTEERING,2107,282347.650,02000000,471d,15824;INS_ALIGNMENT_COMPLETE,INS_RTKFIXED,37.37059194697,126.72433163028,10.7970,22.3000,-0.1569,0.2242,0.0124,-0.943778320,2.029286352,120.707003262,0.4813,0.3140,0.6303,0.1252,0.1036,0.0771,0.1422,0.1473,4.9596,0f000001,0*cfe1604c\n\tsystem status\tnormal 2 28.000000 0 0\trobot status\t309.716473\t51.241452\t10.797000\t-0.943778\t2.029286\t-30.707003\t0.298000\t0.003000\n\t\n15:25:30.1\tlog_raw\tgps_raw\t\tsystem status\tnormal 2 28.000000 0 0\trobot status\t309.824654\t51.161235\t10.804200\t-1.015962\t1.882683\t-30.753433\t0.303000\t-0.001000\n\t\n15:25:30.6\tlog_raw\tgps_raw\t#INSPVAXA,USB3,0,51.5,FINESTEERING,2107,282348.650,02000000,471d,15824;INS_ALIGNMENT_COMPLETE,INS_RTKFIXED,37.37059036777,126.72433430477,10.8134,22.3000,-0.1636,0.2313,0.0075,-1.033266783,1.805769894,120.739350596,0.4628,0.3038,0.6031,0.1249,0.1034,0.0763,0.1419,0.1472,4.9599,0f000001,0*467420a2\n\tsystem status\tnormal 2 28.000000 0 0\trobot status\t309.953375\t51.066177\t10.813400\t-1.033267\t1.805770\t-30.739351\t0.305000\t0.008000\n\t\n15:25:31.1\tlog_raw\tgps_raw\t\tsystem status\tnormal 2 28.000000 0 0\trobot status\t310.058969\t50.987386\t10.820900\t-1.067789\t1.656083\t-30.787262\t0.298000\t0.004000\n\t\n15:25:31.6\tlog_raw\tgps_raw\t#INSPVAXA,USB3,0,51.5,FINESTEERING,2107,282349.650,02000000,471d,15824;INS_ALIGNMENT_COMPLETE,INS_RTKFIXED,37.37058879299,126.72433694056,10.8279,22.3000,-0.1661,0.2333,0.0109,-1.186914388,1.463198419,120.784374977,0.4532,0.2999,0.5832,0.1247,0.1026,0.0761,0.1414,0.1469,4.9608,0f000001,0*9616f401\n\tsystem status\tnormal 2 28.000000 0 0\trobot status\t310.186849\t50.891392\t10.827900\t-1.186914\t1.463198\t-30.784375\t0.291000\t-0.005000\n\t\n15:25:32.1\tlog_raw\tgps_raw\t#INSPVAXA,USB3,0,52.5,FINESTEERING,2107,282350.150,02000000,471d,15824;INS_ALIGNMENT_COMPLETE,INS_RTKFIXED,37.37058797901,126.72433827202,10.8352,22.3000,-0.1763,0.2301,0.0086,-1.055570073,1.334834507,120.760295852,0.4480,0.2986,0.5686,0.1241,0.1011,0.0762,0.1408,0.1465,4.9619,0f000001,0*f726bccb\n\tsystem status\tnormal 2 28.000000 0 0\trobot status\t310.304788\t50.801048\t10.835200\t-1.055570\t1.334835\t-30.760296\t0.299000\t-0.001000\n\t\n15:25:32.6\tlog_raw\tgps_raw\t#INSPVAXA,USB3,0,52.5,FINESTEERING,2107,282350.650,02000000,471d,15824;INS_ALIGNMENT_COMPLETE,INS_RTKFIXED,37.37058716740,126.72433957539,10.8417,22.3000,-0.1740,0.2264,0.0121,-0.872298800,1.208067122,120.805643727,0.4480,0.2986,0.5686,0.1241,0.1011,0.0762,0.1408,0.1465,4.9619,0f000001,0*1bc0a6ef\n\tsystem status\tnormal 2 28.000000 0 0\trobot status\t310.420238\t50.710968\t10.841700\t-0.872299\t1.208067\t-30.805644\t0.296000\t-0.003000\n\t\n15:25:33.1\tlog_raw\tgps_raw\t#INSPVAXA,USB3,0,53.5,FINESTEERING,2107,282351.150,02000000,471d,15824;INS_ALIGNMENT_COMPLETE,INS_RTKFIXED,37.37058636021,126.72434089175,10.8474,22.3000,-0.1737,0.2293,0.0134,-0.911883774,0.960654196,120.863326137,0.4480,0.2986,0.5686,0.1241,0.1011,0.0762,0.1408,0.1465,4.9619,0f000001,0*f3ef71b8\n\tsystem status\tnormal 2 28.000000 0 0\trobot status\t310.536839\t50.621378\t10.847400\t-0.911884\t0.960654\t-30.863326\t0.298000\t0.004000\n\t\n15:25:33.6\tlog_raw\tgps_raw\t#INSPVAXA,USB3,0,53.5,FINESTEERING,2107,282351.650,02000000,471d,15824;INS_ALIGNMENT_COMPLETE,INS_RTKFIXED,37.37058558937,126.72434215471,10.8538,22.3000,-0.1759,0.2200,0.0154,-0.934777564,1.004148344,120.872982319,0.4480,0.2986,0.5686,0.1241,0.1011,0.0762,0.1408,0.1465,4.9619,0f000001,0*31170c67\n\tsystem status\tnormal 2 28.000000 0 0\trobot status\t310.648710\t50.535822\t10.853800\t-0.934778\t1.004148\t-30.872982\t0.298000\t0.002000\n\t\n15:25:34.1\tlog_raw\tgps_raw\t#INSPVAXA,USB3,0,53.0,FINESTEERING,2107,282352.150,02000000,471d,15824;INS_ALIGNMENT_COMPLETE,INS_RTKFIXED,37.37058479579,126.72434342427,10.8616,22.3000,-0.1887,0.2204,0.0143,-0.790488347,0.999839674,120.821997376,0.4480,0.2986,0.5686,0.1241,0.1011,0.0762,0.1408,0.1465,4.9619,0f000001,0*9c9f2292\n\tsystem status\tnormal 2 28.000000 0 0\trobot status\t310.761166\t50.447743\t10.861600\t-0.790488\t0.999840\t-30.821997\t0.299000\t0.003000\n\t\n15:25:34.6\tlog_raw\tgps_raw\t#INSPVAXA,USB3,0,53.0,FINESTEERING,2107,282352.650,02000000,471d,15824;INS_ALIGNMENT_COMPLETE,INS_RTKFIXED,37.37058401212,126.72434466825,10.8699,22.3000,-0.1898,0.2115,0.0109,-0.691065939,1.126816556,120.801550290,0.4480,0.2986,0.5686,0.1241,0.1011,0.0762,0.1408,0.1465,4.9619,0f000001,0*dfeeaeca\n\tsystem status\tnormal 2 28.000000 0 0\trobot status\t310.871355\t50.360763\t10.869900\t-0.691066\t1.126817\t-30.801550\t0.294000\t0.013000\n\t\n15:25:35.1\tlog_raw\tgps_raw\t#INSPVAXA,USB3,0,54.5,FINESTEERING,2107,282353.150,02000000,471d,15824;INS_ALIGNMENT_COMPLETE,INS_RTKFIXED,37.37058321062,126.72434596398,10.8773,22.3000,-0.1742,0.2198,0.0094,-0.675574846,1.167497971,120.763135201,0.5451,0.3682,0.6457,0.1338,0.1065,0.0809,0.1421,0.1478,4.9659,0f000001,0*3ed9f220\n\tsystem status\tnormal 2 28.000000 0 0\trobot status\t310.986129\t50.271805\t10.877300\t-0.675575\t1.167498\t-30.763135\t0.278000\t0.042000\n\t\n15:25:35.6\tlog_raw\tgps_raw\t#INSPVAXA,USB3,0,54.5,FINESTEERING,2107,282353.650,02000000,471d,15824;INS_ALIGNMENT_COMPLETE,INS_RTKFIXED,37.37058240140,126.72434728277,10.8821,22.3000,-0.1762,0.2174,0.0139,-0.658240149,1.464684464,120.605097651,0.5451,0.3682,0.6457,0.1338,0.1065,0.0809,0.1421,0.1478,4.9659,0f000001,0*55075841\n\tsystem status\tnormal 2 28.000000 0 0\trobot status\t311.102945\t50.181990\t10.882100\t-0.658240\t1.464684\t-30.605098\t0.293000\t0.014000\n\t\n15:25:36.1\tlog_raw\tgps_raw\t#INSPVAXA,USB3,0,46.0,FINESTEERING,2107,282354.150,02000000,471d,15824;INS_ALIGNMENT_COMPLETE,INS_RTKFIXED,37.37058158517,126.72434860573,10.8883,22.3000,-0.1761,0.2236,0.0096,-0.460607316,1.517794635,120.410253165,0.4992,0.3307,0.6168,0.1257,0.0997,0.0788,0.1413,0.1466,4.9674,0f000001,0*75609bcc\n\tsystem status\tnormal 2 28.000000 0 0\trobot status\t311.220131\t50.091396\t10.888300\t-0.460607\t1.517795\t-30.410253\t0.287000\t0.028000\n\t\n15:25:36.6\tlog_raw\tgps_raw\t#INSPVAXA,USB3,0,46.0,FINESTEERING,2107,282354.650,02000000,471d,15824;INS_ALIGNMENT_COMPLETE,INS_RTKFIXED,37.37058081600,126.72434991701,10.8934,22.3000,-0.1786,0.2176,0.0091,-0.549619810,1.573012469,120.242291746,0.4992,0.3307,0.6168,0.1257,0.0997,0.0788,0.1413,0.1466,4.9674,0f000001,0*21503aba\n\tsystem status\tnormal 2 28.000000 0 0\trobot status\t311.336282\t50.006026\t10.893400\t-0.549620\t1.573012\t-30.242292\t0.244000\t0.088000\n\t\n15:25:37.1\tlog_raw\tgps_raw\t#INSPVAXA,USB3,0,52.5,FINESTEERING,2107,282355.150,02000000,471d,15824;INS_ALIGNMENT_COMPLETE,INS_RTKFIXED,37.37058003617,126.72435122954,10.8990,22.3000,-0.1704,0.2109,0.0104,-0.583465901,1.528119993,119.981024145,0.4739,0.3119,0.5957,0.1220,0.0977,0.0777,0.1410,0.1462,4.9689,0f000001,0*126057fe\n\tsystem status\tnormal 2 28.000000 0 0\trobot status\t311.452544\t49.919473\t10.899000\t-0.583466\t1.528120\t-29.981024\t0.242000\t0.080000\n\t\n15:25:37.6\tlog_raw\tgps_raw\t#INSPVAXA,USB3,0,52.5,FINESTEERING,2107,282355.650,02000000,471d,15824;INS_ALIGNMENT_COMPLETE,INS_RTKFIXED,37.37057924767,126.72435254533,10.9045,22.3000,-0.1778,0.2238,0.0059,-0.556149260,1.423178014,119.692620317,0.4739,0.3119,0.5957,0.1220,0.0977,0.0777,0.1410,0.1462,4.9689,0f000001,0*50fd9e16\n\tsystem status\tnormal 2 28.000000 0 0\trobot status\t311.569094\t49.831957\t10.904500\t-0.556149\t1.423178\t-29.692620\t0.284000\t0.024000\n\t\n15:25:38.1\tlog_raw\tgps_raw\t#INSPVAXA,USB3,0,50.5,FINESTEERING,2107,282356.150,02000000,471d,15824;INS_ALIGNMENT_COMPLETE,INS_RTKFIXED,37.37057847739,126.72435384843,10.9119,22.3000,-0.1686,0.2211,0.0250,-0.610838091,1.352028935,119.375016734,0.4594,0.3023,0.5798,0.1203,0.0972,0.0771,0.1409,0.1459,4.9699,0f000001,0*f72577eb\n\tsystem status\tnormal 2 28.000000 0 0\trobot status\t311.684521\t49.746463\t10.911900\t-0.610838\t1.352029\t-29.375017\t0.248000\t0.079000\n\t\n15:25:38.6\tlog_raw\tgps_raw\t#INSPVAXA,USB3,0,50.5,FINESTEERING,2107,282356.650,02000000,471d,15824;INS_ALIGNMENT_COMPLETE,INS_RTKFIXED,37.37057772160,126.72435517265,10.9178,22.3000,-0.1723,0.2271,0.0230,-0.636591933,1.172282791,119.120900603,0.4594,0.3023,0.5798,0.1203,0.0972,0.0771,0.1409,0.1459,4.9699,0f000001,0*423d8117\n\tsystem status\tnormal 2 27.900000 0 0\trobot status\t311.801818\t49.662578\t10.917800\t-0.636592\t1.172283\t-29.120901\t0.246000\t0.082000\n\t\n15:25:39.1\tlog_raw\tgps_raw\t#INSPVAXA,USB3,0,52.0,FINESTEERING,2107,282357.150,02000000,471d,15824;INS_ALIGNMENT_COMPLETE,INS_RTKFIXED,37.37057699183,126.72435647012,10.9247,22.3000,-0.1655,0.2123,0.0266,-0.635674987,1.199232102,118.840756157,0.4503,0.2976,0.5676,0.1194,0.0970,0.0768,0.1408,0.1458,4.9705,0f000001,0*6596f8d2\n\tsystem status\tnormal 2 28.000000 0 0\trobot status\t311.916746\t49.581580\t10.924700\t-0.635675\t1.199232\t-28.840756\t0.241000\t0.093000\n\t\n15:25:39.6\tlog_raw\tgps_raw\t#INSPVAXA,USB3,0,52.0,FINESTEERING,2107,282357.650,02000000,471d,15824;INS_ALIGNMENT_COMPLETE,INS_RTKFIXED,37.37057627543,126.72435778684,10.9314,22.3000,-0.1654,0.2174,0.0126,-0.648643975,1.318562977,118.602215065,0.4503,0.2976,0.5676,0.1194,0.0970,0.0768,0.1408,0.1458,4.9705,0f000001,0*56e0c8f4\n\tsystem status\tnormal 2 28.000000 0 0\trobot status\t312.033379\t49.502067\t10.931400\t-0.648644\t1.318563\t-28.602215\t0.336000\t-0.047000\n\t\n15:25:40.1\tlog_raw\tgps_raw\t#INSPVAXA,USB3,0,49.0,FINESTEERING,2107,282358.150,02000000,471d,15824;INS_ALIGNMENT_COMPLETE,INS_RTKFIXED,37.37057556621,126.72435909816,10.9380,22.3000,-0.1614,0.2140,0.0160,-0.816236405,1.456902249,118.427735128,0.4453,0.2956,0.5586,0.1188,0.0967,0.0767,0.1406,0.1456,4.9710,0f000001,0*b637b657\n\tsystem status\tnormal 2 28.000000 0 0\trobot status\t312.149533\t49.423350\t10.938000\t-0.816236\t1.456902\t-28.427735\t0.250000\t0.087000\n\t\n15:25:40.6\tlog_raw\tgps_raw\t#INSPVAXA,USB3,0,49.0,FINESTEERING,2107,282358.650,02000000,471d,15824;INS_ALIGNMENT_COMPLETE,INS_RTKFIXED,37.37057483953,126.72436042274,10.9431,22.3000,-0.1620,0.2072,0.0216,-0.840006247,1.481756490,118.251827857,0.4453,0.2956,0.5586,0.1188,0.0967,0.0767,0.1406,0.1456,4.9710,0f000001,0*14500fa5\n\tsystem status\tnormal 2 28.000000 0 0\trobot status\t312.266862\t49.342695\t10.943100\t-0.840006\t1.481756\t-28.251828\t0.263000\t0.061000\n\t\n15:25:41.1\tlog_raw\tgps_raw\t#INSPVAXA,USB3,0,50.0,FINESTEERING,2107,282359.150,02000000,471d,15824;INS_ALIGNMENT_COMPLETE,INS_RTKFIXED,37.37057411290,126.72436171376,10.9480,22.3000,-0.1710,0.2086,0.0288,-0.732849795,1.756620997,118.132387326,0.4424,0.2949,0.5520,0.1182,0.0959,0.0768,0.1404,0.1455,4.9710,0f000001,0*33ffa9dc\n\tsystem status\tnormal 2 28.000000 0 0\trobot status\t312.381219\t49.262046\t10.948000\t-0.732850\t1.756621\t-28.132387\t0.248000\t0.084000\n\t\n15:25:41.6\tlog_raw\tgps_raw\t#INSPVAXA,USB3,0,50.0,FINESTEERING,2107,282359.650,02000000,471d,15824;INS_ALIGNMENT_COMPLETE,INS_RTKFIXED,37.37057338322,126.72436305467,10.9529,22.3000,-0.1728,0.2229,0.0180,-0.801068797,1.536454287,118.115818478,0.4424,0.2949,0.5520,0.1182,
